vi "_Add Ability Log.vi"(7 "Done? (Starting)":bool) -> ()   [LabVIEW 2022 SP3, in "FlexBlocks Support.lvlib"]
uses:
  FlexBlocks Support.lvlib
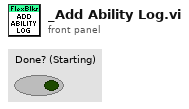
[diagram p1: front panel]
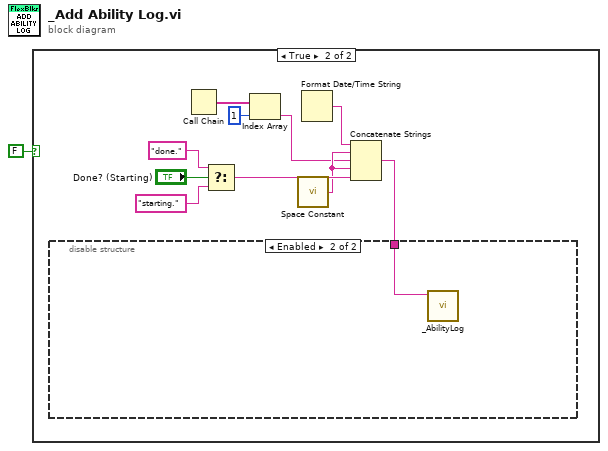
[diagram p0: block diagram]
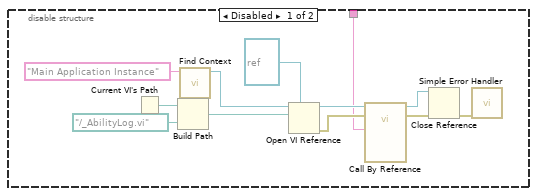
[diagram p3: hidden frame]
diagram:
  n1 = case shown="True" FALSE {
    frame False {
    }
    frame True {
      n2 = Call Chain() -> (call chain=w8:string[])
      n3 = Select(t="done.", s="Done? (Starting)", f="starting.") -> (s? t:f=w6:string)
      n4 = Index Array(array=w8, index=1) -> (element=w3:string)
      n5 = call <vilib>:"Space Constant.vi"() -> ("String"=w5:string)
      n6 = Format Date/Time String() -> (date/time string=w4:string)  [unwired: 3 in]
      n7 = Concatenate Strings(w4, w5, w3, w5, w6) -> (w2:string)
      n8 = disable-structure shown="Enabled" {
        disable-tunnel: w2 -> [w15 w24]
        frame Disabled {
          n9 = Current VI's Path() -> (path=w23:path)
          n10 = Build Path(base path=w23, name or relative path=path "../_AbilityLog.vi") -> (appended path=w21:path)
          n11 = call "Find Context.vi"("Name"="Main Application Instance") -> ("App"=w19:refnum<vi>)  [unwired: 9 in, 1 out]
          n12 = Open VI Reference(type specifier VI Refnum (for type only)=refnum<vi> refnum, application reference (local)=w19, vi path=w21) -> (vi reference=w18:refnum<vi>, error out=w17:errorcluster)  [unwired: 3 in]
          n13 = call-by-ref "?"(reference=w18, error in=w17, "Log Entry"=w15) -> (reference out=w13:refnum<vi>, error out=w14:errorcluster)  [unwired: 11 in]
          n14 = Close Reference(reference=w13, error in (no error)=w14) -> (error out=w12:errorcluster)
          n15 = call <vilib>:"Simple Error Handler.vi"("error in (no error)"=w12) -> ()  [unwired: 4 in, 5 out]
        }
        frame Enabled {
          n16 = call "_AbilityLog.vi"("Log Entry"=w24) -> ()  [unwired: 11 in]
        }
      }
    }
  }
